vi "vclTimeToTimestamp.vi"(3 "all rows":dbl[](array[numeric])) -> (0 "before 2009?":bool, 1 "Array":timestamp[](array[timestamp]))   [LabVIEW 2016, in "VCL_2_DSC.lvclass"]
uses:
  VCL_2_DSC.lvclass
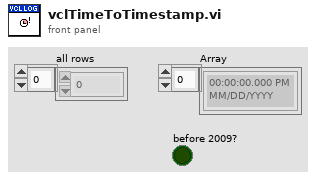
[diagram p1: front panel]
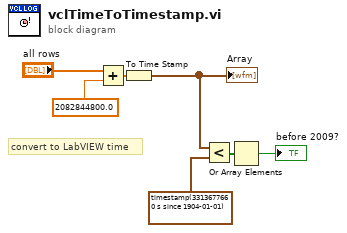
[diagram p0: block diagram]
diagram:
  # "convert to LabVIEW time"
  n1 = Add(x="all rows", y=2082844800.0 ("Numeric 2")) -> (x+y=w7:dbl[])
  n2 = To Time Stamp(1:w7) -> (0:w4:timestamp[])
  "Array" <- w4
  n3 = Less?(x=w4, y=timestamp(3313677660 s since 1904-01-01)) -> (x < y?=w2:bool[])
  n4 = Or Array Elements(Boolean array=w2) -> (logical OR=→"before 2009?":bool)
